vi "uObserver_Set_Policy_Pub.vi"(8 "error in (no error)":errorcluster, 10 "uStringManipulation":refnum<class "uStringManipulation.lvclass">, 11 "uObserver in":refnum<class "uObserver.lvclass">) -> (0 "error out":errorcluster, 3 "uObserver out":refnum<class "uObserver.lvclass">)   [LabVIEW 2021, in "uFramework_pack_uActor.lvlib" / "uObserver.lvclass"]
uses:
  uObserver.lvclass
  Bin/uFramework.lvlibp/uStringManipulation/uStringManipulation.lvclass
  uObserver.lvclass/uObserver.ctl
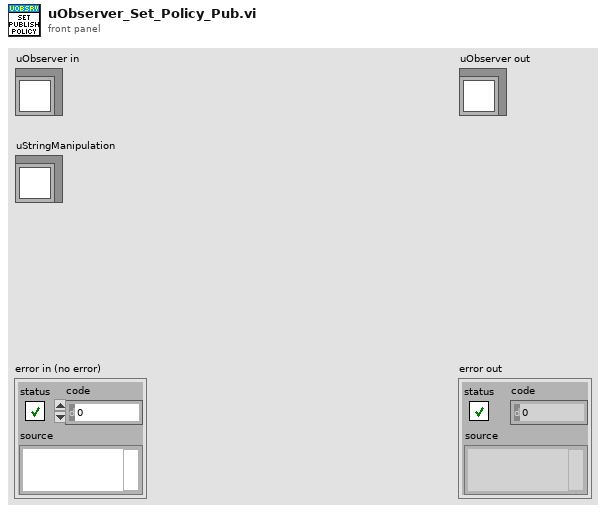
[diagram p1: front panel]
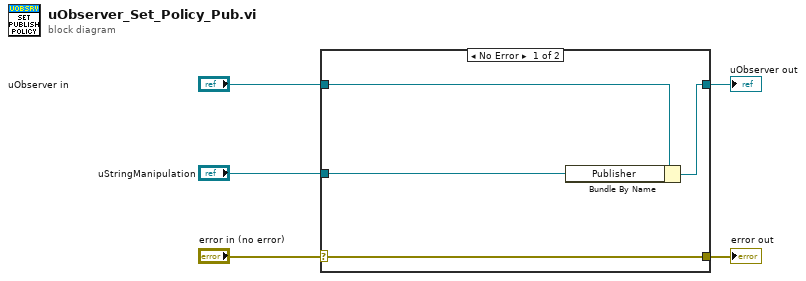
[diagram p0: block diagram]
diagram:
  n1 = case shown="No Error" "error in (no error)" {
    selector: "error in (no error)" -> [w9 w10]
    tunnel: [w9 w10] -> w4
    tunnel: [w7 w11] -> w2
    tunnel: "uObserver in" -> [w8 w11]
    tunnel: "uStringManipulation" -> [w6 _]
    frame No Error {
      n2 = Bundle By Name(cluster=w8, "Publisher"=w6) -> (w7:refnum<class "uObserver.lvclass">)
    }
    frame Error {
    }
  }
  "error out" <- w4
  "uObserver out" <- w2
